vi "RemoteDCPowerSession_CallCloseMeasurementLinkSessionWithDetachBehavior_RemoteSessionDetached.vi"(8 "error in (no error)":errorcluster) -> (0 "error out":errorcluster, 2 "result":string, 3 "pass":bool)   [LabVIEW 2020, in "MeasurementServerTests.lvlib"]
uses:
  MeasurementServerTests.lvlib
  Runtime/MeasurementLink niDCPower/Instrument/Instrument.lvclass
  Runtime/MeasurementLink Instrument/IInstrument/Close Session Behavior.ctl
  Runtime/MeasurementLink Instrument/IInstrument/IInstrument.lvclass
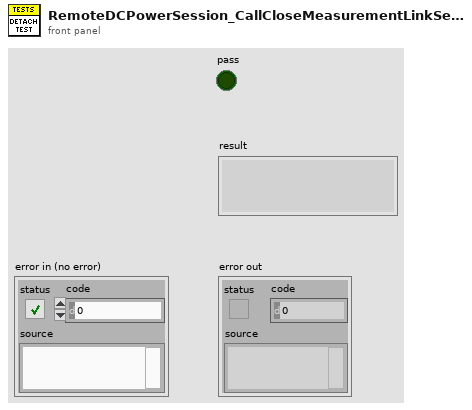
[diagram p1: front panel]
types:
  T1 = typedef "MeasurementLink Instrument.lvlib/IInstrument.lvclass/Close Session Behavior.ctl" = enum16{"Close Session", "Detach Session"}
  T2 = typedef "MeasurementLink Instrument.lvlib/IInstrument.lvclass/Remote Connection Options.ctl" = cluster{"session name":string, "address":string, "port":u32}
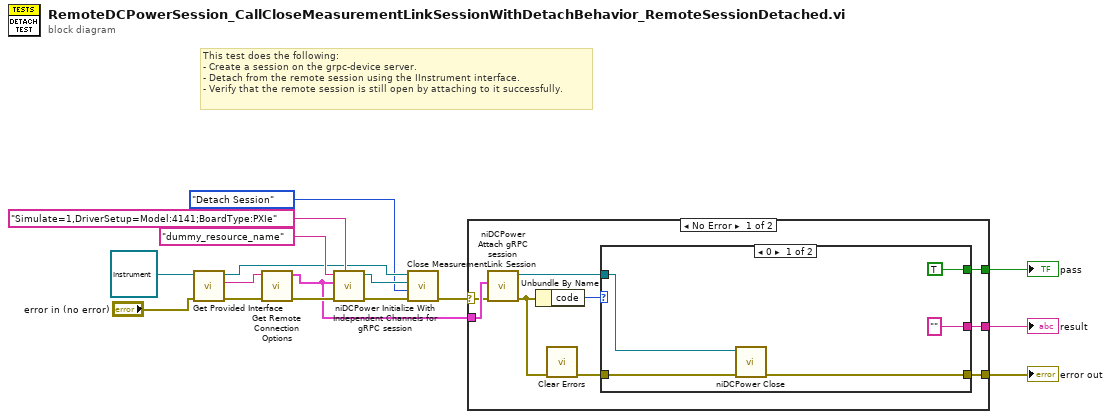
[diagram p0: block diagram]
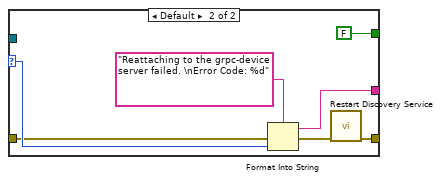
[diagram p2: hidden frame]
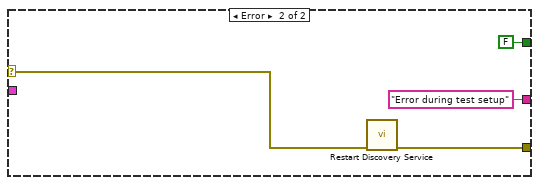
[diagram p3: hidden frame]
diagram:
  # "This test does the following:\n- Create a session on the grpc-device server.\n- Detach from the remote session using the IInstrument interface.\n- Verify that the remote session is still open by attaching to it successfully."
  n1 = call-dynamic "Get Provided Interface.vi"("error in (no error)"="error in (no error)", "instrument in"=refnum<class "Instrument.lvclass"> refnum ("MeasurementLink niDCPower.lvlib:Instrument.lvclass")) -> ("error out"=w13:errorcluster, "provided interface"=w12:string, "instrument out"=w9:refnum<class "Instrument.lvclass">)  [unwired: 7 in]
  n2 = call "Get Remote Connection Options.vi"("error in (no error)"=w13, "provided interface"=w12) -> ("error out"=w15:errorcluster, "remote connection options"=w1:T2)  [unwired: 8 in]
  n3 = call <instrlib>:"niDCPower Initialize With Independent Channels for gRPC session.vi"("option string"="Simulate=1,DriverSetup=Model:4141;BoardType:PXIe", "error in (no error)"=w15, "gRPC options"=w1, "resource name"="dummy_resource_name") -> ("error out"=w10:errorcluster, "instrument handle out"=w8:refnum<k15>)  [unwired: 6 in]
  n4 = call-dynamic "Close MeasurementLink Session.vi"("error in (no error)"=w10, "close session behavior"=Close_Session_Behavior."Detach Session", "session in"=w8, "instrument in"=w9) -> ("error out"=w2:errorcluster)  [unwired: 7 in]
  n5 = case shown="No Error" w2 {
    selector: w2 -> [w24 w39]
    tunnel: w1 -> [w25 _]
    tunnel: [w19 w38] -> w3
    tunnel: [w23 FALSE] -> w5
    tunnel: [w18 "Error during test setup" ("f")] -> w4
    frame No Error {
      n6 = call <instrlib>:"niDCPower Attach gRPC session.vi"("error in (no error)"=w24, "gRPC options"=w25) -> ("error out"=w21:errorcluster, "instrument handle out"=w17:refnum<k15>)  [unwired: 8 in]
      n7 = Unbundle By Name(w21) -> ("code"=w22:i32)
      n8 = call <vilib>:"Clear Errors.vi"("error in (no error)"=w21) -> ("error out"=w20:errorcluster)  [unwired: 5 in, 1 out]
      n9 = case shown="0" w22 {
        selector: w22 -> [_ w36]
        tunnel: ["" ("f") w35] -> w18
        tunnel: [TRUE FALSE] -> w23
        tunnel: w20 -> [w28 w33]
        tunnel: [w27 w31] -> w19
        tunnel: w17 -> [w26 _]
        frame 0 {
          n10 = call <instrlib>:"niDCPower Close.vi"("error in (no error)"=w28, "instrument handle"=w26) -> ("error out"=w27:errorcluster)  [unwired: 9 in]
        }
        frame Default {
          n11 = Format Into String(format string="Reattaching to the grpc-device server failed. \nError Code: %d" ("f"), error in=w33, w36) -> (resulting string=w35:string, error out=w32:errorcluster)  [unwired: 1 in]
          n12 = call "Restart Discovery Service.vi"("error in"=w32) -> ("error out"=w31:errorcluster)  [unwired: 10 in]
        }
      }
    }
    frame Error {
      n13 = call "Restart Discovery Service.vi"("error in"=w39) -> ("error out"=w38:errorcluster)  [unwired: 10 in]
    }
  }
  "error out" <- w3
  "pass" <- w5
  "result" <- w4
